vi "Table-Set column selection.vi"(6 "Selection length (i.e. Number of rows)":i32, 8 "error in (no error)":errorcluster, 9 "Index of column to select":i32, 10 "Index of row to select":i32, 11 "Table in":refnum<vi>) -> (0 "error out":errorcluster, 3 "Table out":refnum<vi>)   [LabVIEW 2013]
uses:
  <vilib>/Utility/miscctls.llb/LVRowAndColumnTypeDef.ctl
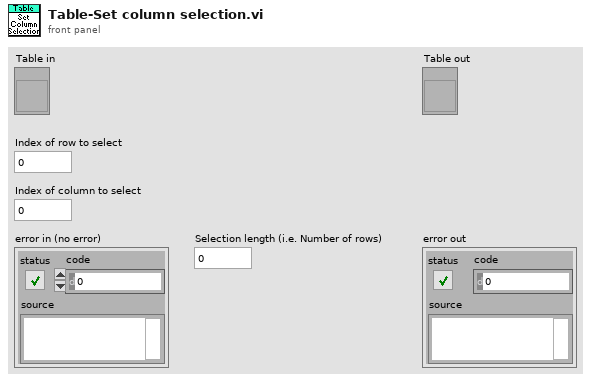
[diagram p1: front panel]
types:
  T1 = typedef "LVRowAndColumnTypeDef.ctl" = cluster{"Row":i32, "Column":i32}
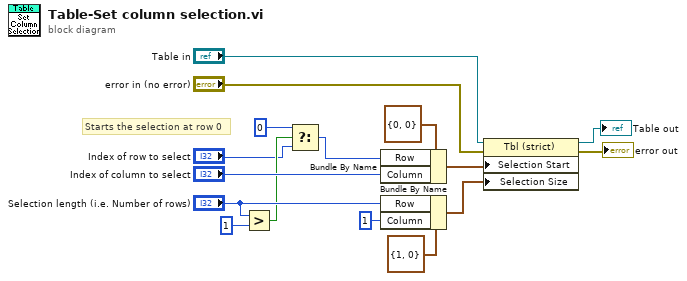
[diagram p0: block diagram]
diagram:
  # "Starts the selection at row 0"
  n1 = Greater?(x="Selection length (i.e. Number of rows)", y=1) -> (0:w4:bool)
  n2 = Select(t=0, s=w4, f="Index of row to select") -> (s? t:f=w2:i32)
  n3 = Bundle By Name(cluster=T1 {"Row"=0, "Column"=0} ("Selection Start"), "Row"=w2, "Column"="Index of column to select") -> (w12:T1)
  n4 = Bundle By Name(cluster=T1 {"Row"=1, "Column"=0} ("Selection Size"), "Row"="Selection length (i.e. Number of rows)", "Column"=1) -> (w13:T1)
  n5 = property on="Property Node" class="Tbl (strict)"(reference="Table in", error in="error in (no error)", "Selection Start"=w12, "Selection Size"=w13) -> (reference out=→"Table out":refnum<vi>, error out=→"error out":errorcluster)
